vi "compute_all.vi"(4 "ItemNames":string[][](array[string]), 5 "additional vol. [ml]":dbl, 6 "pipette vol. [ml]":dbl, 7 "calibration vol. [ml]":dbl, 8 "temperature [°C]":dbl, 9 "humidity [%]":dbl, 10 "pressure [mbar]":dbl) -> (0 "mols":dbl, 1 "Array":string[][](array[string]), 2 "pout":dbl, 3 "wvp":dbl)   [LabVIEW 2013]
doc: "Berechnung des:\n- dry pressure im Volumen der Cal\n- mole im Volumen der Cal\n- CalAmounts im Volumen der Cal und der Pipette"
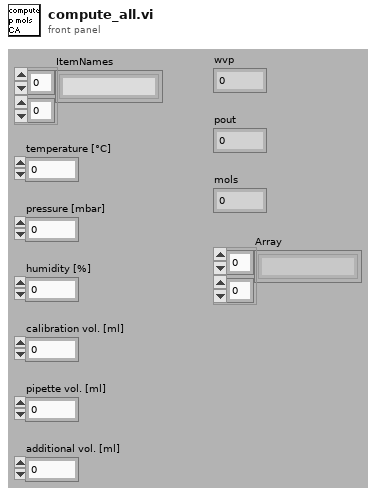
[diagram p1: front panel]
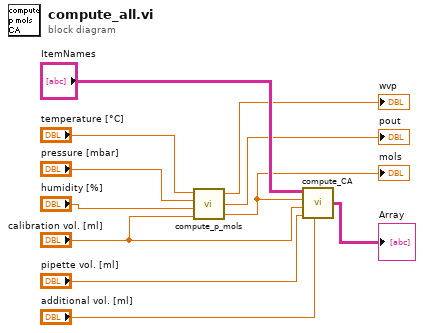
[diagram p0: block diagram]
diagram:
  n1 = call "compute_p_mols.vi"("calibration vol. [ml]"="calibration vol. [ml]", "humidity [%]"="humidity [%]", "pressure [mbar]"="pressure [mbar]", "temperature [°C]"="temperature [°C]") -> ("mols"=w9:dbl, "pout"=→"pout":dbl, "wvp"=→"wvp":dbl)
  "mols" <- w9
  n2 = call "compute_CA.vi"("additional vol. [ml]"="additional vol. [ml]", "pipette vol. [ml]"="pipette vol. [ml]", "calibration vol. [ml]"="calibration vol. [ml]", "mols in Cal-volume"=w9, "ItemNames"="ItemNames") -> ("Array"=→"Array":string[][])  [unwired: 1 in]
